vi "Shader.vi"(1 "输入":u32[][](array[numeric]), 2 "颜色":u32) -> (0 "输出":u32[][](array[numeric]))   [LabVIEW 2016]
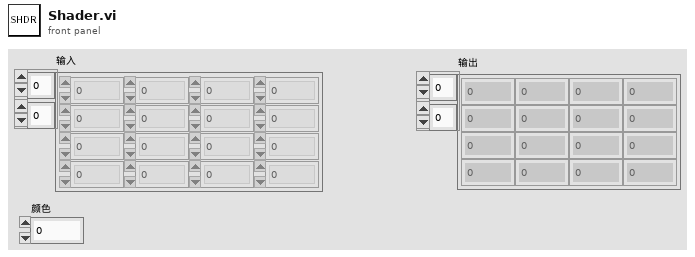
[diagram p1: front panel]
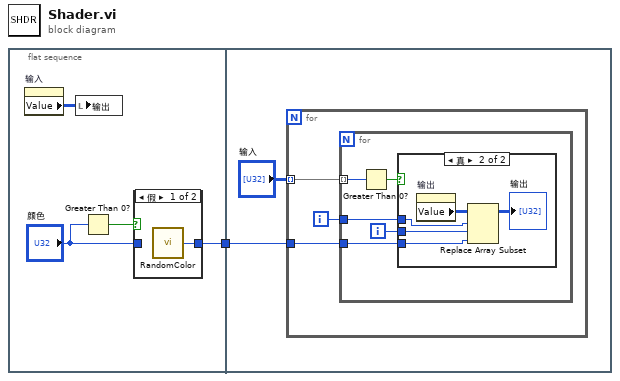
[diagram p0: block diagram]
diagram:
  n1 = flat-sequence {
    tunnel: [w2] -> w1
    tunnel: w1 -> [w8]
    frame #0 {
      n2 = property on="输入" class="Arr (严格)"() -> ("Value"=w5:u32[][])  [unwired: 2 in, 2 out]
      n3 = local write "输出"(w5) -> ()
      n4 = Greater Than 0?(x="颜色") -> (x > 0?=w4:bool)
      n5 = case shown="假" w4 {
        tunnel: [w6 w7] -> w2
        tunnel: "颜色" -> [_ w7]
        frame False {
          n6 = call "RandomColor.vi"() -> ("数值"=w6:u32)
        }
        frame True {
        }
      }
    }
    frame #1 {
      n7 = for {
        tunnel: "输入" -> [w12] mode=indexing
        tunnel: w8 -> [w10]
        i -> [w11]
        n8 = for {
          tunnel: w12 -> [w17] mode=indexing
          tunnel: w11 -> [w16]
          tunnel: w10 -> [w13]
          i -> [w15]
          n9 = Greater Than 0?(x=w17) -> (x > 0?=w14:bool)
          n10 = case shown="真" w14 {
            tunnel: w16 -> [_ w21]
            tunnel: w15 -> [_ w20]
            tunnel: w13 -> [_ w18]
            frame False {
            }
            frame True {
              n11 = property on="输出" class="Arr (严格)"() -> ("Value"=w22:u32[][])  [unwired: 2 in, 2 out]
              n12 = Replace Array Subset(array=w22, new element=w18, index (row)=w21, index (col)=w20) -> (→"输出":u32[][])
            }
          }
        }
      }
    }
  }
